vi "Get_Current_Scan_client.vi"(0 "singleChannel":string, 1 "multipleChannels":string[](array[string])) -> (2 "Ch Description Array":T1[](array[typedef]) {"Duty" format="%016b"; "D" format="%#_5g"; "C" format="%#_5g"; "B" format="%#_5g"; "A" format="%#_5g"}, 3 "String values":string[](array[string]), 4 "Numerical Values":dbl[](array[numeric]) format="%.9f", 5 "firstString":string)   [LabVIEW 2020]
uses:
  Sub VIs/ADAM Controls/Ch_description_ADAM.ctl
  Sub VIs/ADAM Controls/Module_type_ADAM.ctl
  Sub VIs/ADAM Controls/Function_ADAM.ctl
  Sub VIs/ADAM Controls/Channel_State.ctl
  Sub VIs/ADAM Controls/Calib_type_ADAM.ctl
  Sub VIs/ADAM Controls/Address.ctl
  Anemometry/Anemometry Sub Vis/Controls/Global_mode.ctl
  Anemometry/Anemometry Sub Vis/Globals/Preference_global.vi
panel:
  out "firstValue":dbl
  in  "server type":refnum<vi>
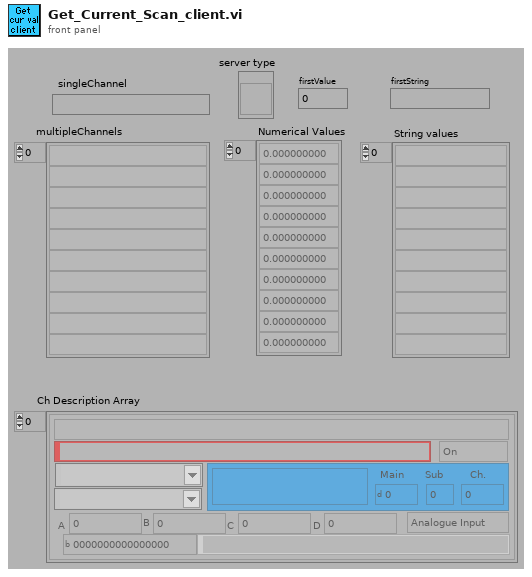
[diagram p1: front panel]
types:
  T1 = typedef "Ch_description_ADAM.ctl" = cluster{"Ch Name":string, "Type":T2, "Function":T3, "Ch State":T4, "Calibration type":T5, "A":dbl, "B":dbl, "C":dbl, "D":dbl, "Comments":string, "Address":T6, "String":string, "Duty":u16}
  T2 = typedef "Module_type_ADAM.ctl" = string
  T3 = typedef "Function_ADAM.ctl" = enum16{"Analogue Input", "Digital Input", "Event counter", "Event rate", "Analogue Output", "Digital Output", "Relay Output"}
  T4 = typedef "Channel_State.ctl" = enum16{"On", "Off", "Always On", "Always Off"}
  T5 = typedef "Calib_type_ADAM.ctl" = string
  T6 = typedef "Address.ctl" = cluster{"Main":i32, "Ch.":i32, "Sub":i32, "Port Name":string}
  T7 = typedef "Server_Comms.ctl" = enum16{"Do Not Link To Server", "Server Link Healthy"}
  T8 = typedef "Global_mode.ctl" = enum16{"Read Global", "Load Global From File", "Write Global to File"}
  T9 = typedef "Update_scan_value.ctl" = cluster{"Channel Name":string, "New Value":dbl}
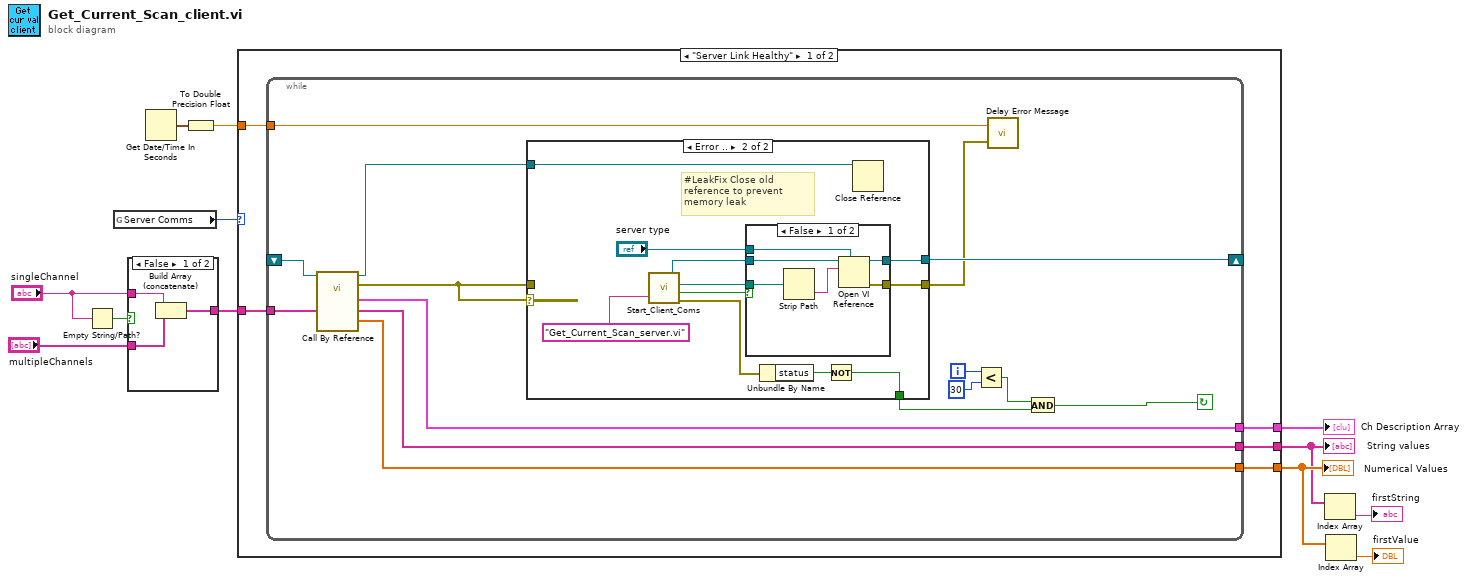
[diagram p0: block diagram]
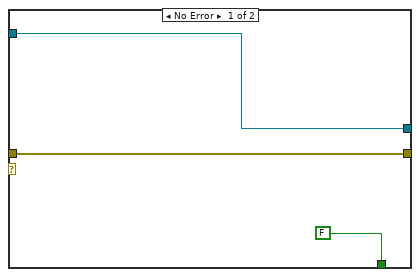
[diagram p3: hidden frame]
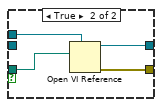
[diagram p4: hidden frame]
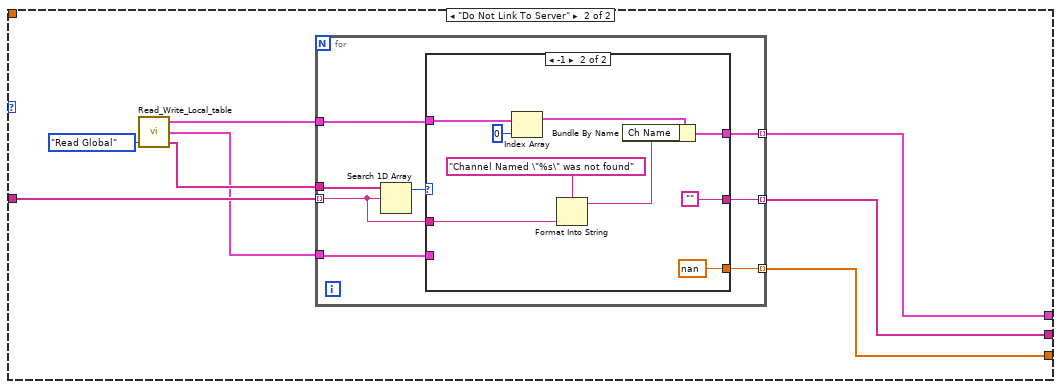
[diagram p5: hidden frame]
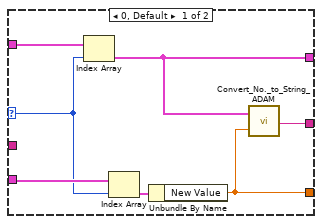
[diagram p6: hidden frame]
diagram:
  n1 = Empty String/Path?(string/path="singleChannel") -> (empty?=w6:bool)
  n2 = global read "Preference_global.vi" "Server Comms"() -> (w12:T7)
  n3 = case shown="False" w6 {
    tunnel: "multipleChannels" -> [w15 w16]
    tunnel: [w14 w16] -> w7
    tunnel: "singleChannel" -> [w13 _]
    frame False {
      n4 = Build Array (concatenate)(w13, w15) -> (w14:string[])
    }
    frame True {
    }
  }
  n5 = Get Date/Time In Seconds() -> (seconds since 1Jan1904=w9:timestamp)
  n6 = To Double Precision Float(number=w9) -> (double precision float=w8:dbl)
  n7 = case shown="\"Server Link Healthy\"" w12 {
    tunnel: w7 -> [w21 w66]
    tunnel: [w18 w61] -> w10
    tunnel: [w20 w64] -> w3
    tunnel: [w19 w63] -> w4
    tunnel: w8 -> [w17 _]
    frame "Server Link Healthy" {
      n8 = while {
        tunnel: [w29] -> w19
        tunnel: [w30] -> w20
        tunnel: w21 -> [w34]
        shift-left: _ -> [w36]
        shift-right: [w32] -> _
        tunnel: [w28] -> w18
        tunnel: w17 -> [w24]
        i -> [w31]
        stop <- w35 continue-if-true
        n9 = call-by-ref "Call By Reference"(reference=w36, "Desired Channels"=w34) -> (reference out=w33:refnum<vi>, error out=w23:errorcluster, "Ch Description Array"=w28:T1[], "String values"=w30:string[], "Numerical Values"=w29:dbl[])  [unwired: 1 in]
        n10 = case shown="Error .." w23 {
          tunnel: [w38 w46] -> w32
          tunnel: [w39 w44] -> w25
          tunnel: w23 -> [w39 _]
          tunnel: w33 -> [w38 w43]
          tunnel: [FALSE w40] -> w22
          frame No Error {
          }
          frame Error {
            # "#LeakFix Close old reference to prevent memory leak"
            n11 = call "Start_Client_Coms.vi"("VI name to run on server"="Get_Current_Scan_server.vi") -> ("LabVIEW application reference"=w48:refnum<vi>, "Checked VI name"=w49:path, "Local Call"=w47:bool, "Error cluster"=w42:errorcluster)  [unwired: 1 in]
            n12 = case shown="False" w47 {
              tunnel: [w54 w60] -> w46
              tunnel: "server type" -> [w53 w59]
              tunnel: w49 -> [w52 w58]
              tunnel: w48 -> [w51 _]
              tunnel: [w55 w57] -> w44
              frame False {
                n13 = Strip Path(path=w52) -> (name=w56:string)  [unwired: 1 out]
                n14 = Open VI Reference(type specifier VI Refnum (for type only)=w53, application reference (local)=w51, vi path=w56) -> (vi reference=w54:refnum<vi>, error out=w55:errorcluster)  [unwired: 1 in, 2 out]
              }
              frame True {
                n15 = Open VI Reference(type specifier VI Refnum (for type only)=w59, vi path=w58) -> (vi reference=w60:refnum<vi>, error out=w57:errorcluster)  [unwired: 1 in, 3 out]
              }
            }
            n16 = Unbundle By Name(w42) -> ("status"=w41:bool)
            n17 = Not(x=w41) -> (.not. x?=w40:bool)
            n18 = Close Reference(reference=w43) -> ()  [unwired: 1 in, 1 out]
          }
        }
        n19 = Less?(x=w31, y=30) -> (x < y?=w27:bool)
        n20 = call "Delay Error Message.vi"("error in (no error)"=w25, "Seconds since 1904"=w24) -> ()  [unwired: 2 in]
        n21 = And(x=w27, y=w22) -> (x .and. y?=w35:bool)
      }
    }
    frame "Do Not Link To Server" {
      n22 = call "Read_Write_Local_table.vi"("Mode"=Global_mode."Read Global") -> ("Ch Names"=w67:string[], "Ch Values Out"=w62:T9[], "Channels Descriptions Out"=w65:T1[])  [unwired: 2 in]
      n23 = for {
        tunnel: w67 -> [w76]
        tunnel: w66 -> [w69] mode=indexing
        tunnel: w65 -> [w74]
        tunnel: [w73] -> w61 mode=indexing
        tunnel: [w72] -> w64 mode=indexing
        tunnel: [w71] -> w63 mode=indexing
        tunnel: w62 -> [w70]
        n24 = Search 1D Array(1D array=w76, element=w69) -> (index of element=w75:i32)  [unwired: 1 out]
        n25 = case shown="-1" w75 {
          selector: w75 -> [w77 _]
          tunnel: w74 -> [w83 w91]
          tunnel: [w80 w89] -> w73
          tunnel: [w78 ""] -> w72
          tunnel: [w79 nan] -> w71
          tunnel: w70 -> [w82 _]
          tunnel: w69 -> [_ w86]
          frame 0, Default {
            n26 = Index Array(array=w83, index=w77) -> (element=w80:T1)
            n27 = Index Array(array=w82, index=w77) -> (element=w81:T9)
            n28 = Unbundle By Name(w81) -> ("New Value"=w79:dbl)
            n29 = call "Convert_No._to_String_ADAM.vi"("Input number"=w79, "Ch Description"=w80) -> ("Output sting"=w78:string)
          }
          frame -1 {
            n30 = Index Array(array=w91, index=0 ("Index")) -> (element=w90:T1)
            n31 = Format Into String(format string="Channel Named \"%s\" was not found" ("Format String"), w86) -> (resulting string=w84:string)  [unwired: 2 in, 1 out]
            n32 = Bundle By Name(cluster=w90, "Ch Name"=w84) -> (w89:T1)
          }
        }
      }
    }
  }
  "Ch Description Array" <- w10
  "String values" <- w3
  "Numerical Values" <- w4
  n33 = Index Array(array=w3) -> (element=→"firstString":string)  [unwired: 1 in]
  n34 = Index Array(array=w4) -> (element=→"firstValue":dbl)  [unwired: 1 in]
